vi "Sort Ascending (single).vi"(8 "error in (no error)":errorcluster, 11 "XY-data in":cluster{"X-array":dbl[], "Y-array":dbl[]}) -> (0 "error out":errorcluster, 3 "XY-data out":cluster{"X-array":dbl[], "Y-array":dbl[]} {"Y-array" format="%.2p"; "X-array" format="%.2p"})   [LabVIEW 2016, in "xy_utilities.lvlib"]
uses:
  xy_utilities.lvlib
  <vilib>/Analysis/NI_AALPro.lvlib
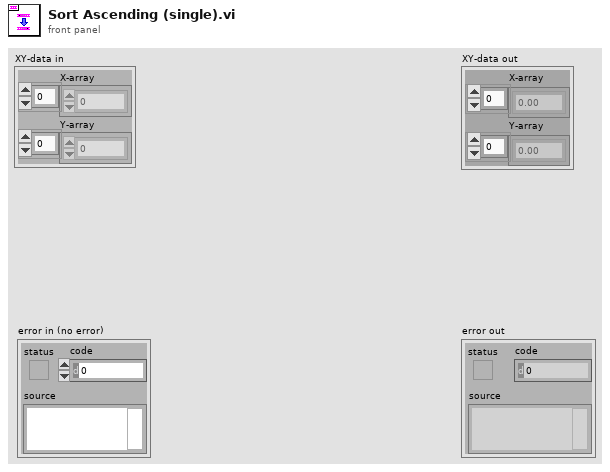
[diagram p1: front panel]
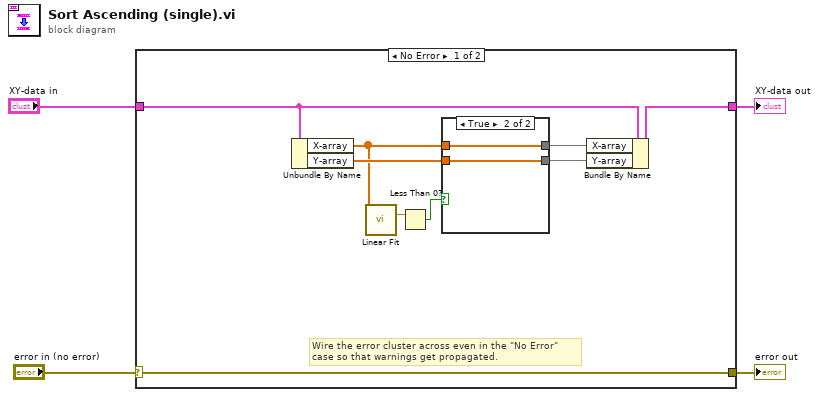
[diagram p0: block diagram]
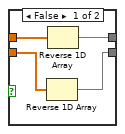
[diagram p2: hidden frame]
diagram:
  n1 = case shown="No Error" "error in (no error)" {
    selector: "error in (no error)" -> [w13 w21]
    tunnel: [w13 w21] -> w3
    tunnel: "XY-data in" -> [w12 w20]
    tunnel: [w11 w20] -> w1
    frame No Error {
      # "Wire the error cluster across even in the \"No Error\"\ncase so that warnings get propagated."
      n2 = Unbundle By Name(w12) -> ("X-array"=w7:dbl[], "Y-array"=w10:dbl[])
      n3 = call <vilib>:"Linear Fit.vi"("Y"=w7) -> ("slope"=w6:dbl)  [unwired: 10 in, 4 out]
      n4 = Less Than 0?(x=w6) -> (x < 0?=w5:bool)
      n5 = case shown="True" w5 {
        tunnel: w7 -> [w17 w19]
        tunnel: w10 -> [w16 w18]
        tunnel: [w15 w18] -> w9
        tunnel: [w14 w19] -> w8
        frame False {
          n6 = Reverse 1D Array(array=w16) -> (reversed array=w15:dbl[])
          n7 = Reverse 1D Array(array=w17) -> (reversed array=w14:dbl[])
        }
        frame True {
        }
      }
      n8 = Bundle By Name(cluster=w12, "X-array"=w8, "Y-array"=w9) -> (w11:cluster{"X-array":dbl[], "Y-array":dbl[]})
    }
    frame Error {
    }
  }
  "error out" <- w3
  "XY-data out" <- w1
